vi "Get.vi"(8 "error in (no error)":errorcluster, 11 "AbstractData in":refnum<class "AbstractData.lvclass">) -> (0 "error out":errorcluster, 2 "Data":variant, 3 "AbstractData out":refnum<class "AbstractData.lvclass">)   [LabVIEW 2014, in "AbstractData.lvclass"]
uses:
  AbstractData.lvclass
  AbstractData.lvclass/AbstractData.ctl
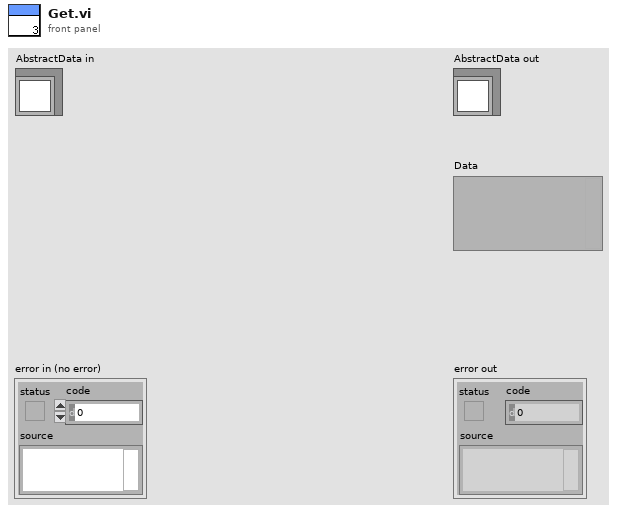
[diagram p1: front panel]
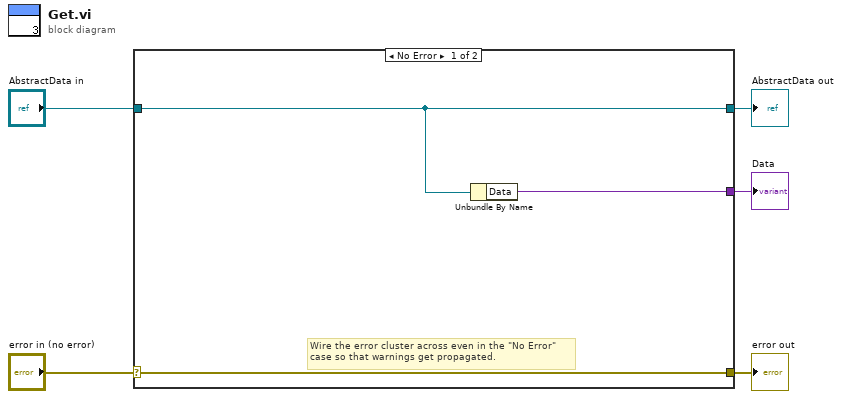
[diagram p0: block diagram]
diagram:
  n1 = case shown="No Error" "error in (no error)" {
    selector: "error in (no error)" -> [w8 w10]
    tunnel: [w8 w10] -> w4
    tunnel: [w6 w9] -> w2
    tunnel: "AbstractData in" -> [w6 w9]
    tunnel: [w7 _] -> w1
    frame No Error {
      # "Wire the error cluster across even in the \"No Error\"\ncase so that warnings get propagated."
      n2 = Unbundle By Name(w6) -> ("Data"=w7:variant)
    }
    frame Error {
    }
  }
  "error out" <- w4
  "AbstractData out" <- w2
  "Data" <- w1
